vi "Read y.vi"(8 "error in (no error)":errorcluster, 11 "Vector2 in":refnum<class "Vector2.lvclass">) -> (0 "error out":errorcluster, 2 "y":sgl, 3 "Vector2 out":refnum<class "Vector2.lvclass">)   [LabVIEW 2022 SP3, in "Vector2.lvclass"]
uses:
  Vector2.lvclass
  Vector2.lvclass/Vector2.ctl
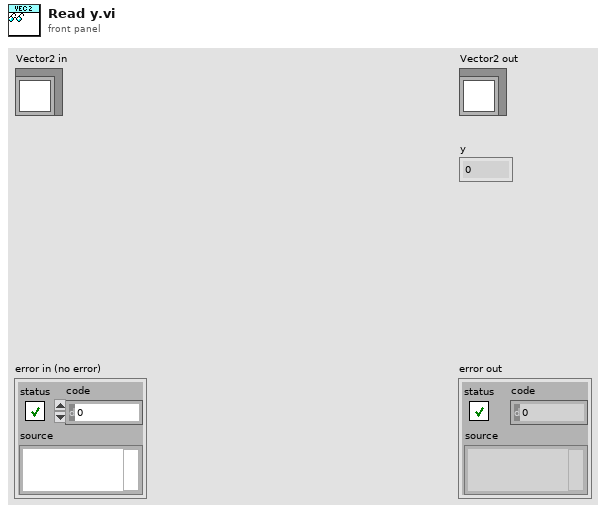
[diagram p1: front panel]
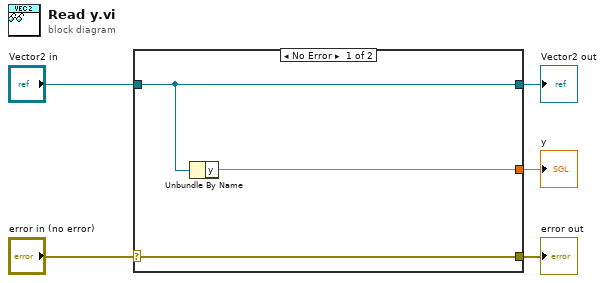
[diagram p0: block diagram]
diagram:
  n1 = case shown="No Error" "error in (no error)" {
    selector: "error in (no error)" -> [w8 w9]
    tunnel: [w8 w9] -> w4
    tunnel: [w7 w10] -> w2
    tunnel: "Vector2 in" -> [w7 w10]
    tunnel: [w6 _] -> w1
    frame No Error {
      n2 = Unbundle By Name(w7) -> ("y"=w6:sgl)
    }
    frame Error {
    }
  }
  "error out" <- w4
  "Vector2 out" <- w2
  "y" <- w1
